vi "VocAging.vi"(0 "time at OC (min)":sgl=10.0, 1 "Device Code":i32=21, 2 "ID":i32=1, 3 "Channel":u8(ring) items=["1", "2", "3", "4", "5", "6", "7", "8", "9", "10", "11", "12", "13", "14", "15", "16"], 4 "instance":i32, 5 "Record_every_dT (s)":sgl=1.0, 7 "record every dE (V)":sgl=0.2, 8 "device area (cm2)":dbl=0.16 caption="Time Target (s)", 9 "Save Data":bool, 11 "error in (no error)":errorcluster, 12 "start time":timestamp, 14 "AgingFile":path=path "C:/EC-Lab Development Package/Examples/Labview/V12/DefaultAging") -> (6 "AverageVoc":dbl, 15 "error out":errorcluster)   [LabVIEW 2020]
doc: "The Open Circuit Voltage technique consists of a period during which no potantial or current is applied to the working electrode.\nThis VI contain others sub VIs.\nIn general,in this VI, the first thing to do is to start by establishing the connection with the instrument defined by its IP adress, then load the firmware in the channel selected, get the information on the plugged channels, load protocol on a channel, start/stop the protocol, retreive data and draw the graph."
uses:
  ActiveArray.vi
  <vilib>/Utility/file.llb/Write Delimited Spreadsheet (DBL).vi
  IntensityTemperature.vi
panel:
  out "finished":bool
  in  "Draw":enum16{"Ewe(t)", "Ece(t)"}(ring)
  out "Number of points":i32
  out "Data 100":dbl[][](array[numeric]) format="%.2f"
  in  "stop":bool
  out "XY Graph":cluster{"Data 100":dbl[], "Data 100":dbl[]}(graph)
  in  "OCV Parameters":T1={"Rest_time_T"=1.0, "Record_every_dE"=0.01, "Record_every_dT"=0.01, "E_Range"=3, "em"=1, "ce"=0, "tb"=0.0001} {"tb" min=2e-05 max=1 format="%^_3e"; "ce" items=["Standard", "CE to ground"]; "E_Range" items=["±2.5V", "±5V", "±10V", "Auto"]; "Record_every_dT" min=0 format="%.2e"; "Record_every_dE" min=0 max=100 format="%.4f"; "Rest_time_T" min=0 format="%.2f"}
  # "Voc Aging"
  # "Rest for time tr( s)"
  # "Record every dEr (V)"
  # "And at least every dtr (s)"
  # "E range"
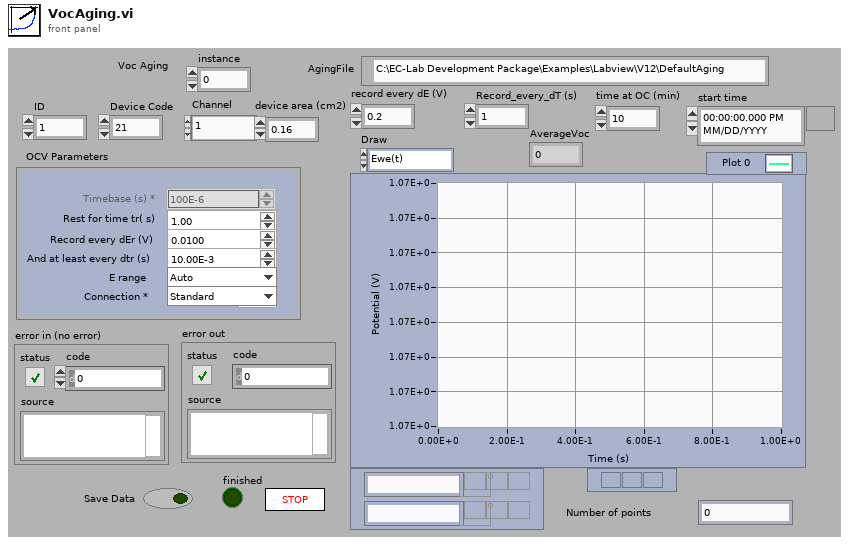
[diagram p1: front panel]
types:
  T1 = cluster{"Rest_time_T":sgl, "Record_every_dE":sgl, "Record_every_dT":sgl, "E_Range":u16, "em":u16, "ce":u16, "tb":sgl}
  T2 = cluster{"Label":string, "type":i32, "valeur":u32, "index":i32}[]
  T3 = cluster{"IRQskipped":i32, "NbRaws":i32, "NbCols":i32, "Technique Index":i32, "TechniqueID":i32, "PrcessIndex":i32, "loop":i32, "StartTime":dbl, "MuxPad":i32}
  T4 = cluster{"State":i32, "MemFilled":i32, "TimeBase":sgl, " Ewe":sgl, " EweRangeMin":sgl, " EweRangeMax":sgl, "Ece":sgl, "EceRangeMin":sgl, "EceRangeMax":sgl, "Eoverflow":i32, "I":sgl, "IRange":i32, "Ioverflow":i32, "ElapsedTime":sgl, "Freq":sgl, "Rcomp":sgl, "Saturation":sgl, "OptErr":i32, "OptPos":i32}
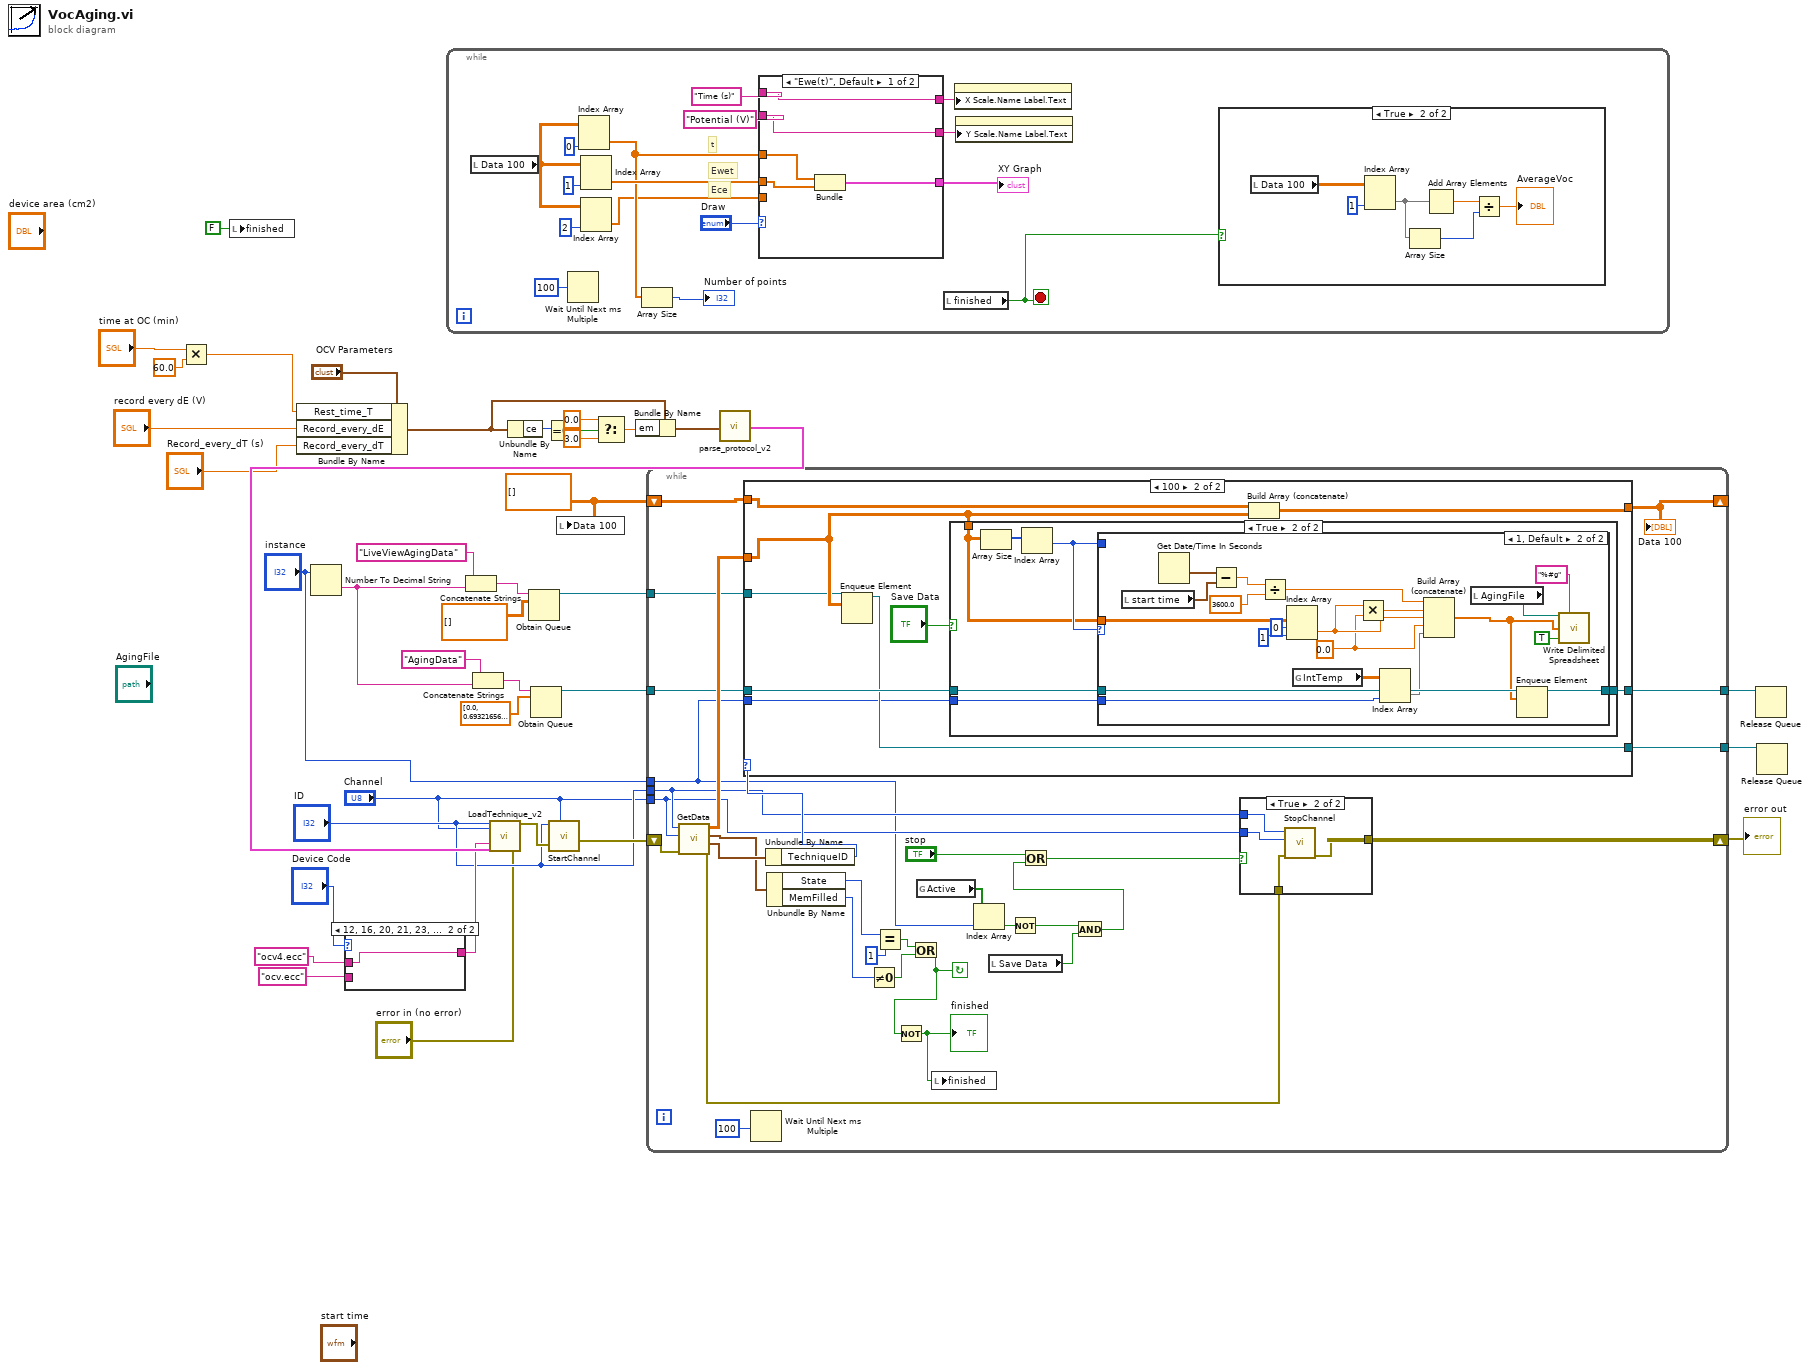
[diagram p0: block diagram]
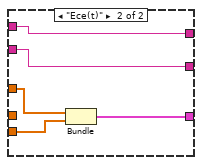
[diagram p8: hidden frame]
diagram:
  w28 = dbl[][] []
  n1 = Multiply(x="time at OC (min)", y=sgl 60.0) -> (x*y=w15:sgl)
  n2 = local write "finished"(FALSE ("finished")) -> ()
  n3 = Bundle By Name(cluster="OCV Parameters", "Rest_time_T"=w15, "Record_every_dE"="record every dE (V)", "Record_every_dT"="Record_every_dT (s)") -> (w20:T1)
  n4 = Number To Decimal String(number="instance") -> (decimal integer string=w13:string)  [unwired: 1 in]
  n5 = case shown="12, 16, 20, 21, 23, 27" "Device Code" {
    tunnel: "ocv.ecc" ("FName") -> [w39 _]
    tunnel: [w39 w40] -> w25
    tunnel: "ocv4.ecc" ("FName") -> [_ w40]
    frame Default {
    }
    frame 12, 16, 20, 21, 23, 27 {
    }
  }
  n6 = while {
    stop <- w41 stop-if-true
    # "Ece"
    # "Ewet"
    # "t"
    n7 = local read "Data 100"() -> (w52:dbl[][])
    n8 = Wait Until Next ms Multiple(millisecond multiple=u32 100) -> ()  [unwired: 1 out]
    n9 = Index Array(array=w52, index (col)=0 ("Index")) -> (element=w45:dbl[])  [unwired: 1 in]
    n10 = Index Array(array=w52, index (col)=1 ("Index")) -> (element=w46:dbl[])  [unwired: 1 in]
    n11 = Index Array(array=w52, index (col)=2 ("indice désactivé (col)")) -> (element=w44:dbl[])  [unwired: 1 in]
    n12 = Array Size(array=w45) -> (size(s)=→"Number of points":i32)
    n13 = case shown="\"Ewe(t)\", Default" "Draw" {
      tunnel: "Time (s)" ("Y Scale.Name Label.Text") -> [w67 w72]
      tunnel: [w67 w72] -> w49
      tunnel: "Potential (V)" ("Y Scale.Name Label.Text") -> [w66 w71]
      tunnel: [w66 w71] -> w47
      tunnel: w45 -> [w65 w68]
      tunnel: w46 -> [w64 _]
      tunnel: w44 -> [_ w70]
      tunnel: [w63 w69] -> w42
      frame "Ewe(t)", Default {
        n14 = Bundle("Data 100"=w65, "Data 100"=w64) -> (w63:cluster{"Data 100":dbl[], "Data 100":dbl[]})  [unwired: 1 in]
      }
      frame "Ece(t)" {
        n15 = Bundle("Data 100"=w68, "Data 100"=w70) -> (w69:cluster{"Data 100":dbl[], "Data 100":dbl[]})  [unwired: 1 in]
      }
    }
    "XY Graph" <- w42
    n16 = local read "finished"() -> (w41:bool)
    n17 = property on="XY Graph" class="XYGraph (strict)"("X Scale.Name Label.Text"=w49) -> ()  [unwired: 2 in, 2 out]
    n18 = property on="XY Graph" class="XYGraph (strict)"("Y Scale.Name Label.Text"=w47) -> ()  [unwired: 2 in, 2 out]
    n19 = case shown="True" w41 {
      frame False {
      }
      frame True {
        n20 = local read "Data 100"() -> (w61:dbl[][])
        n21 = Index Array(array=w61, index (col)=1 ("Index")) -> (element=w60:dbl[])  [unwired: 1 in]
        n22 = Array Size(array=w60) -> (size(s)=w58:i32)
        n23 = Add Array Elements(numeric array=w60) -> (sum=w59:dbl)
        n24 = Divide(x=w59, y=w58) -> (x/y=→"AverageVoc":dbl)
      }
    }
  }
  n25 = Concatenate Strings("LiveViewAgingData" ("name (unnamed)"), w13) -> (w8:string)
  n26 = Concatenate Strings("AgingData" ("name (unnamed)"), w13) -> (w11:string)
  n27 = Unbundle By Name(w20) -> ("ce"=w32:u16)
  n28 = Obtain Queue(name (unnamed)=w8, element data type=sgl[][] []) -> (queue out=w5:refnum<queue>)  [unwired: 3 in, 2 out]
  n29 = Obtain Queue(name (unnamed)=w11, element data type=dbl[] [0.0, 0.6932165634222212, 0.002936372303467471, 0.2869923716049554, 0.0005841850023007069, 0.39914193749427795, 0.001463602161096093, 0.0, 0.0, 0.0, 0.0, 0.0, 0.0, inf] ("appended array 2")) -> (queue out=w4:refnum<queue>)  [unwired: 3 in, 2 out]
  n30 = Equal To 0?(x=w32) -> (x = 0?=w33:bool)
  n31 = local write "Data 100"(w28) -> ()
  n32 = Select(t=0.0, s=w33, f=3.0) -> (s? t:f=w29:dbl)
  n33 = Bundle By Name(cluster=w20, "em"=w29) -> (w34:T1)
  n34 = call "parse_protocol_v2.vi"("Protocol Cluster"=w34) -> ("Params Values"=w35:T2)
  n35 = call "LoadTechnique_v2.vi"("ID"="ID", "Selected Channel"="Channel", "FName"=w25, "Protocol Parameters"=w35, "error in (no error)"="error in (no error)") -> ("error out"=w26:errorcluster)  [unwired: 14 in]
  n36 = call "StartChannel.vi"("error in (no error)"=w26, "Channel"="Channel", "ID"="ID") -> ("error out"=w27:errorcluster)  [unwired: 8 in]
  n37 = while {
    shift-right: [w98] -> w22
    shift-left: w27 -> [w100]
    shift-right: [w82] -> _
    shift-left: w28 -> [w96]
    tunnel: "Channel" -> [w81]
    tunnel: "ID" -> [w90]
    tunnel: w5 -> [w80]
    tunnel: w4 -> [w79]
    tunnel: [w78] -> w3
    tunnel: [w77] -> w2
    tunnel: "instance" -> [w73]
    stop <- w88 continue-if-true
    n38 = call "GetData.vi"("error in (no error)"=w100, "Channel"=w81, "ID"=w90) -> ("error out"=w87:errorcluster, "Data information"=w94:T3, "Current values"=w91:T4, "Data"=w97:dbl[][])  [unwired: 5 in]
    n39 = Wait Until Next ms Multiple(millisecond multiple=u32 100) -> ()  [unwired: 1 out]
    n40 = Unbundle By Name(w94) -> ("TechniqueID"=w95:i32)
    n41 = case shown="100" w95 {
      tunnel: w97 -> [_ w120]
      tunnel: [w111 w118] -> w82
      tunnel: w96 -> [w111 w119]
      tunnel: w80 -> [w110 w117]
      tunnel: w79 -> [w109 w116]
      tunnel: [w109 w115] -> w78
      tunnel: [w110 w114] -> w77
      tunnel: w73 -> [_ w112]
      frame 0, Default {
      }
      frame 100 {
        n42 = Enqueue Element(queue=w117, element=w120) -> (queue out=w114:refnum<queue>)  [unwired: 2 in, 2 out]
        n43 = case shown="True" "Save Data" {
          tunnel: w120 -> [_ w125]
          tunnel: w116 -> [w121 w124]
          tunnel: [w121 w123] -> w115
          tunnel: w112 -> [_ w122]
          frame False {
          }
          frame True {
            n44 = Array Size(array=w125) -> (size(s)=w126:i32[])
            n45 = Index Array(array=w126) -> (element=w127:i32)  [unwired: 1 in]
            n46 = case shown="1, Default" w127 {
              tunnel: w125 -> [_ w138]
              tunnel: w127 -> [_ _]
              tunnel: w124 -> [w128 w137]
              tunnel: [w128 w136] -> w123
              tunnel: w122 -> [_ w134]
              frame 0 {
              }
              frame 1, Default {
                w131 = 0.0 ("y")
                n47 = local read "start time"() -> (w142:timestamp)
                n48 = Get Date/Time In Seconds() -> (seconds since 1Jan1904=w143:timestamp)
                n49 = Subtract(x=w143, y=w142) -> (x-y=w145:dbl)
                n50 = Divide(x=w145, y=3600.0) -> (x/y=w130:dbl)
                n51 = Index Array(array=w138, index (row)=0 ("disabled index (row)"), index (col)=1 ("Index")) -> (element=w139:dbl)
                n52 = global read "IntensityTemperature.vi" "IntTemp"() -> (w135:dbl[][])
                n53 = Multiply(x=w139, y=w131) -> (x*y=w140:dbl)
                n54 = Index Array(array=w135, index (col)=w134) -> (element=w133:dbl[])  [unwired: 1 in]
                n55 = Build Array (concatenate)(w130, w140, w139, w131, w133) -> (w129:dbl[])
                n56 = local read "AgingFile"() -> (w147:path)
                n57 = Enqueue Element(queue=w137, element=w129) -> (queue out=w136:refnum<queue>)  [unwired: 2 in, 2 out]
                n58 = call-poly <vilib>:"Write Delimited Spreadsheet.vi"("file path (dialog if empty)"=w147, "format (%.3f)"="%#g", "1D data"=w129, "append to file? (new file:F)"=TRUE ("append to file? (F)")) -> ()  [unwired: 10 in, 2 out]
              }
            }
          }
        }
        n59 = Build Array (concatenate)(w119, w120) -> (w118:dbl[][])
      }
    }
    "Data 100" <- w82
    n60 = Unbundle By Name(w91) -> ("State"=w93:i32, "MemFilled"=w92:i32)
    n61 = Not Equal To 0?(x=w92) -> (x != 0?=w101:bool)
    n62 = Equal?(x=w93, y=1) -> (x = y?=w102:bool)
    n63 = Or(x=w102, y=w101) -> (x .or. y?=w88:bool)
    n64 = Not(x=w88) -> (.not. x?=w89:bool)
    "finished" <- w89
    n65 = global read "ActiveArray.vi" "Active"() -> (w86:bool[])
    n66 = local write "finished"(w89) -> ()
    n67 = Index Array(array=w86, index=w73) -> (element=w85:bool)
    n68 = local read "Save Data"() -> (w75:bool)
    n69 = Not(x=w85) -> (.not. x?=w76:bool)
    n70 = And(x=w76, y=w75) -> (x .and. y?=w74:bool)
    n71 = Or(x="stop", y=w74) -> (x .or. y?=w84:bool)
    n72 = case shown="True" w84 {
      tunnel: [w104 w108] -> w98
      tunnel: w87 -> [w104 w107]
      tunnel: w81 -> [_ w106]
      tunnel: w90 -> [_ w105]
      frame False {
      }
      frame True {
        n73 = call "StopChannel.vi"("error in (no error)"=w107, "Channel"=w106, "ID"=w105) -> ("error out"=w108:errorcluster)  [unwired: 8 in]
      }
    }
  }
  "error out" <- w22
  n74 = Release Queue(queue=w3) -> ()  [unwired: 2 in, 3 out]
  n75 = Release Queue(queue=w2) -> ()  [unwired: 2 in, 3 out]
